vi "Roller IR Logic Test.vi"() -> ()   [LabVIEW 2013]
uses:
  Robot Code/Rollers/Roller Control.ctl
  Robot Code/Rollers/Roller Mode.ctl
panel:
  in  "Manual Roller Command In":T1
  out "Back Roller":dbl(slide) scale=-1.0..1.0
  out "Front Roller":dbl(slide) scale=-1.0..1.0
  out "Roller Command Out":T1
  in  "stop":bool
  # "Note: change the \"Roller IR Logic.vi\" to use\nthe disabled code (controls for IRs and Timeouts)"
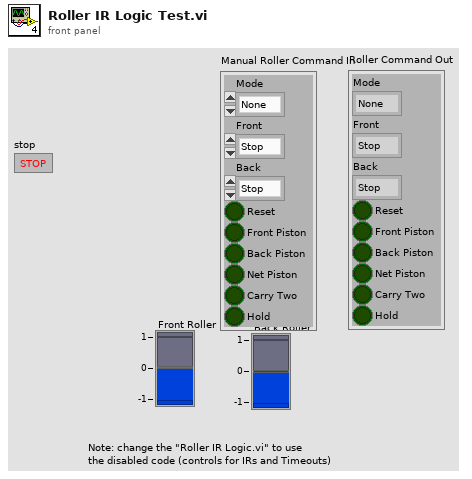
[diagram p1: front panel]
types:
  T1 = typedef "Roller Control.ctl" = cluster{"Mode":T2, "Front":enum16{"Stop", "Forward", "Reverse"}, "Back":enum16{"Stop", "Forward", "Reverse"}, "Reset":bool, "Front Piston":bool, "Back Piston":bool, "Net Piston":bool, "Carry Two":bool, "Hold":bool}
  T2 = typedef "Roller Mode.ctl" = enum16{"None", "Front", "Back", "Both", "Manual"}
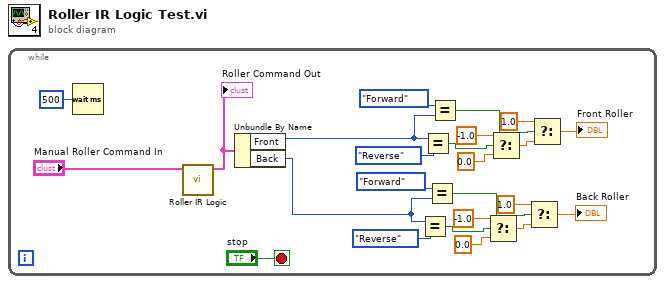
[diagram p0: block diagram]
diagram:
  n1 = while {
    stop <- "stop" stop-if-true
    n2 = Wait (ms)(milliseconds to wait=u32 500) -> ()  [unwired: 1 out]
    n3 = call "Roller IR Logic.vi"("Roller Command In"="Manual Roller Command In") -> ("Roller Command Out"=w22:T1)  [unwired: 10 in]
    "Roller Command Out" <- w22
    n4 = Unbundle By Name(w22) -> ("Front"=w14:enum16{"Stop", "Forward", "Reverse"}, "Back"=w3:enum16{"Stop", "Forward", "Reverse"})
    n5 = Equal?(x=w3, y=enum16{"Stop", "Forward", "Reverse"}."Reverse") -> (x = y?=w6:bool)
    n6 = Equal?(x=w14, y=enum16{"Stop", "Forward", "Reverse"}."Reverse") -> (x = y?=w19:bool)
    n7 = Equal?(x=enum16{"Stop", "Forward", "Reverse"}."Forward" ("y"), y=w3) -> (x = y?=w11:bool)
    n8 = Equal?(x=enum16{"Stop", "Forward", "Reverse"}."Forward" ("y"), y=w14) -> (x = y?=w13:bool)
    n9 = Select(t=-1.0 ("f"), s=w6, f=0.0 ("t")) -> (s? t:f=w9:dbl)
    n10 = Select(t=-1.0 ("f"), s=w19, f=0.0 ("t")) -> (s? t:f=w16:dbl)
    n11 = Select(t=1.0 ("f"), s=w11, f=w9) -> (s? t:f=→"Back Roller":dbl)
    n12 = Select(t=1.0 ("f"), s=w13, f=w16) -> (s? t:f=→"Front Roller":dbl)
  }
